vi "RampUpMKII.vi"() -> ()   [LabVIEW 2010]
panel:
  in  "Right Power In":i8=100
  out "Right Power Out":i8
  in  "# of Samples":sgl=10.0
  in  "Left Power In":i8=100
  out "Left Power out":i8
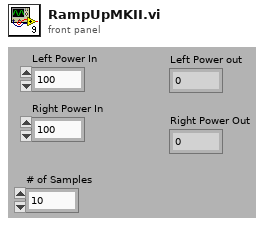
[diagram p1: front panel]
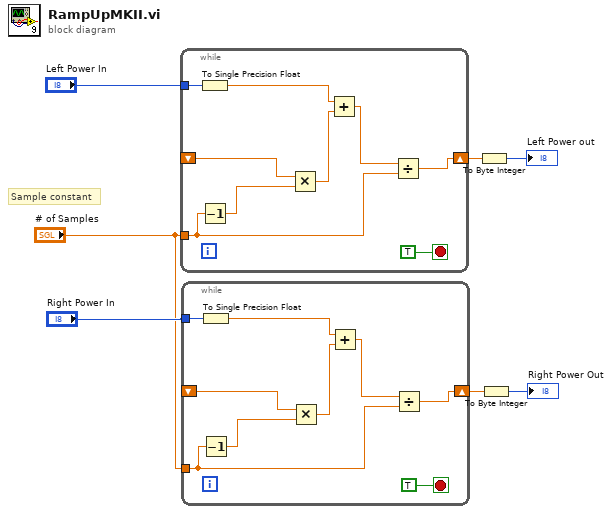
[diagram p0: block diagram]
diagram:
  # "Sample constant"
  n1 = while {
    tunnel: "# of Samples" -> [w11]
    tunnel: "Left Power In" -> [w14]
    shift-right: [w8] -> w6
    shift-left: _ -> [w10]
    stop <- TRUE stop-if-true
    n2 = To Single Precision Float(number=w14) -> (single precision float=w9:sgl)
    n3 = Decrement(x=w11) -> (x-1=w15:sgl)
    n4 = Multiply(x=w10, y=w15) -> (x*y=w13:sgl)
    n5 = Add(x=w9, y=w13) -> (x+y=w12:sgl)
    n6 = Divide(x=w12, y=w11) -> (x/y=w8:sgl)
  }
  n7 = while {
    tunnel: "# of Samples" -> [w20]
    tunnel: "Right Power In" -> [w23]
    shift-right: [w17] -> w1
    shift-left: _ -> [w19]
    stop <- TRUE stop-if-true
    n8 = To Single Precision Float(number=w23) -> (single precision float=w18:sgl)
    n9 = Decrement(x=w20) -> (x-1=w24:sgl)
    n10 = Multiply(x=w19, y=w24) -> (x*y=w22:sgl)
    n11 = Add(x=w18, y=w22) -> (x+y=w21:sgl)
    n12 = Divide(x=w21, y=w20) -> (x/y=w17:sgl)
  }
  n13 = To Byte Integer(number=w6) -> (8bit integer=→"Left Power out":i8)
  n14 = To Byte Integer(number=w1) -> (8bit integer=→"Right Power Out":i8)
